vi "Field Draw Field(circular).vi"(7 "FieldRef":refnum<class "Field.lvclass">=refnum, 8 "new picture in":picture, 9 "Offset":cluster{"Width":dbl, "Height":dbl}, 10 "Scale":dbl) -> (0 "new picture out":picture, 1 "Offset Out":cluster{"Width":dbl, "Height":dbl}, 2 "Scale Out":dbl)   [LabVIEW 2022 SP3]
uses:
  Field_class/Field.lvclass
panel:
  in  "left":i16=1
  in  "rect":T1
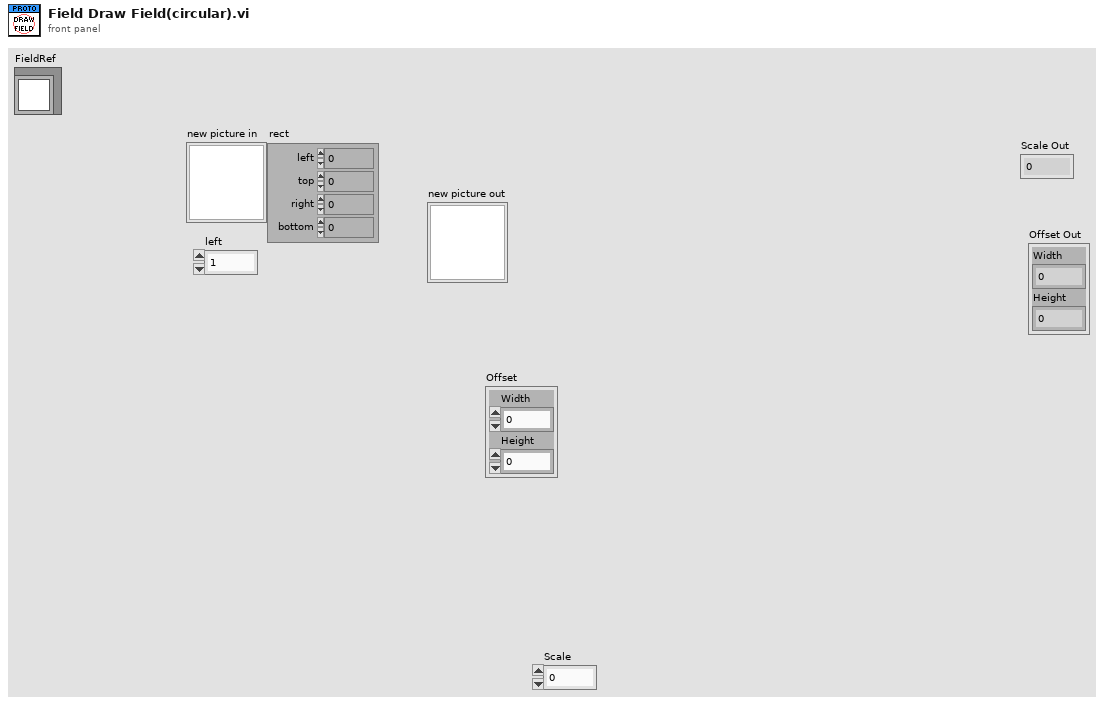
[diagram p1: front panel]
types:
  T1 = cluster{"left":i16, "top":i16, "right":i16, "bottom":i16}
  T2 = cluster{"Width":i16, "Style":enum32{"Solid", "Dash", "Dot", "DashDot", "DashDotDot"}}
  T3 = cluster{"boundary_width":i32, "center_circle_radius":i32, "defense_stretch":i32, "defense_width_or_radius":i32, "field_length":i32, "field_width":i32, "free_kick_from_defense_dist":i32, "goal_depth":i32, "goal_wall_width":i32, "goal_width":i32, "line_width":i32, "penalty_line_from_spot_dist":i32, "penalty_spot_from_field_line_dist":i32, "referee_width":i32}
  T4 = cluster{"boundary_width":dbl, "center_circle_radius":dbl, "defense_stretch":dbl, "defense_width_or_radius":dbl, "field_length":dbl, "field_width":dbl, "free_kick_from_defense_dist":dbl, "goal_depth":dbl, "goal_wall_width":dbl, "goal_width":dbl, "line_width":dbl, "penalty_line_from_spot_dist":dbl, "penalty_spot_from_field_line_dist":dbl, "referee_width":dbl}
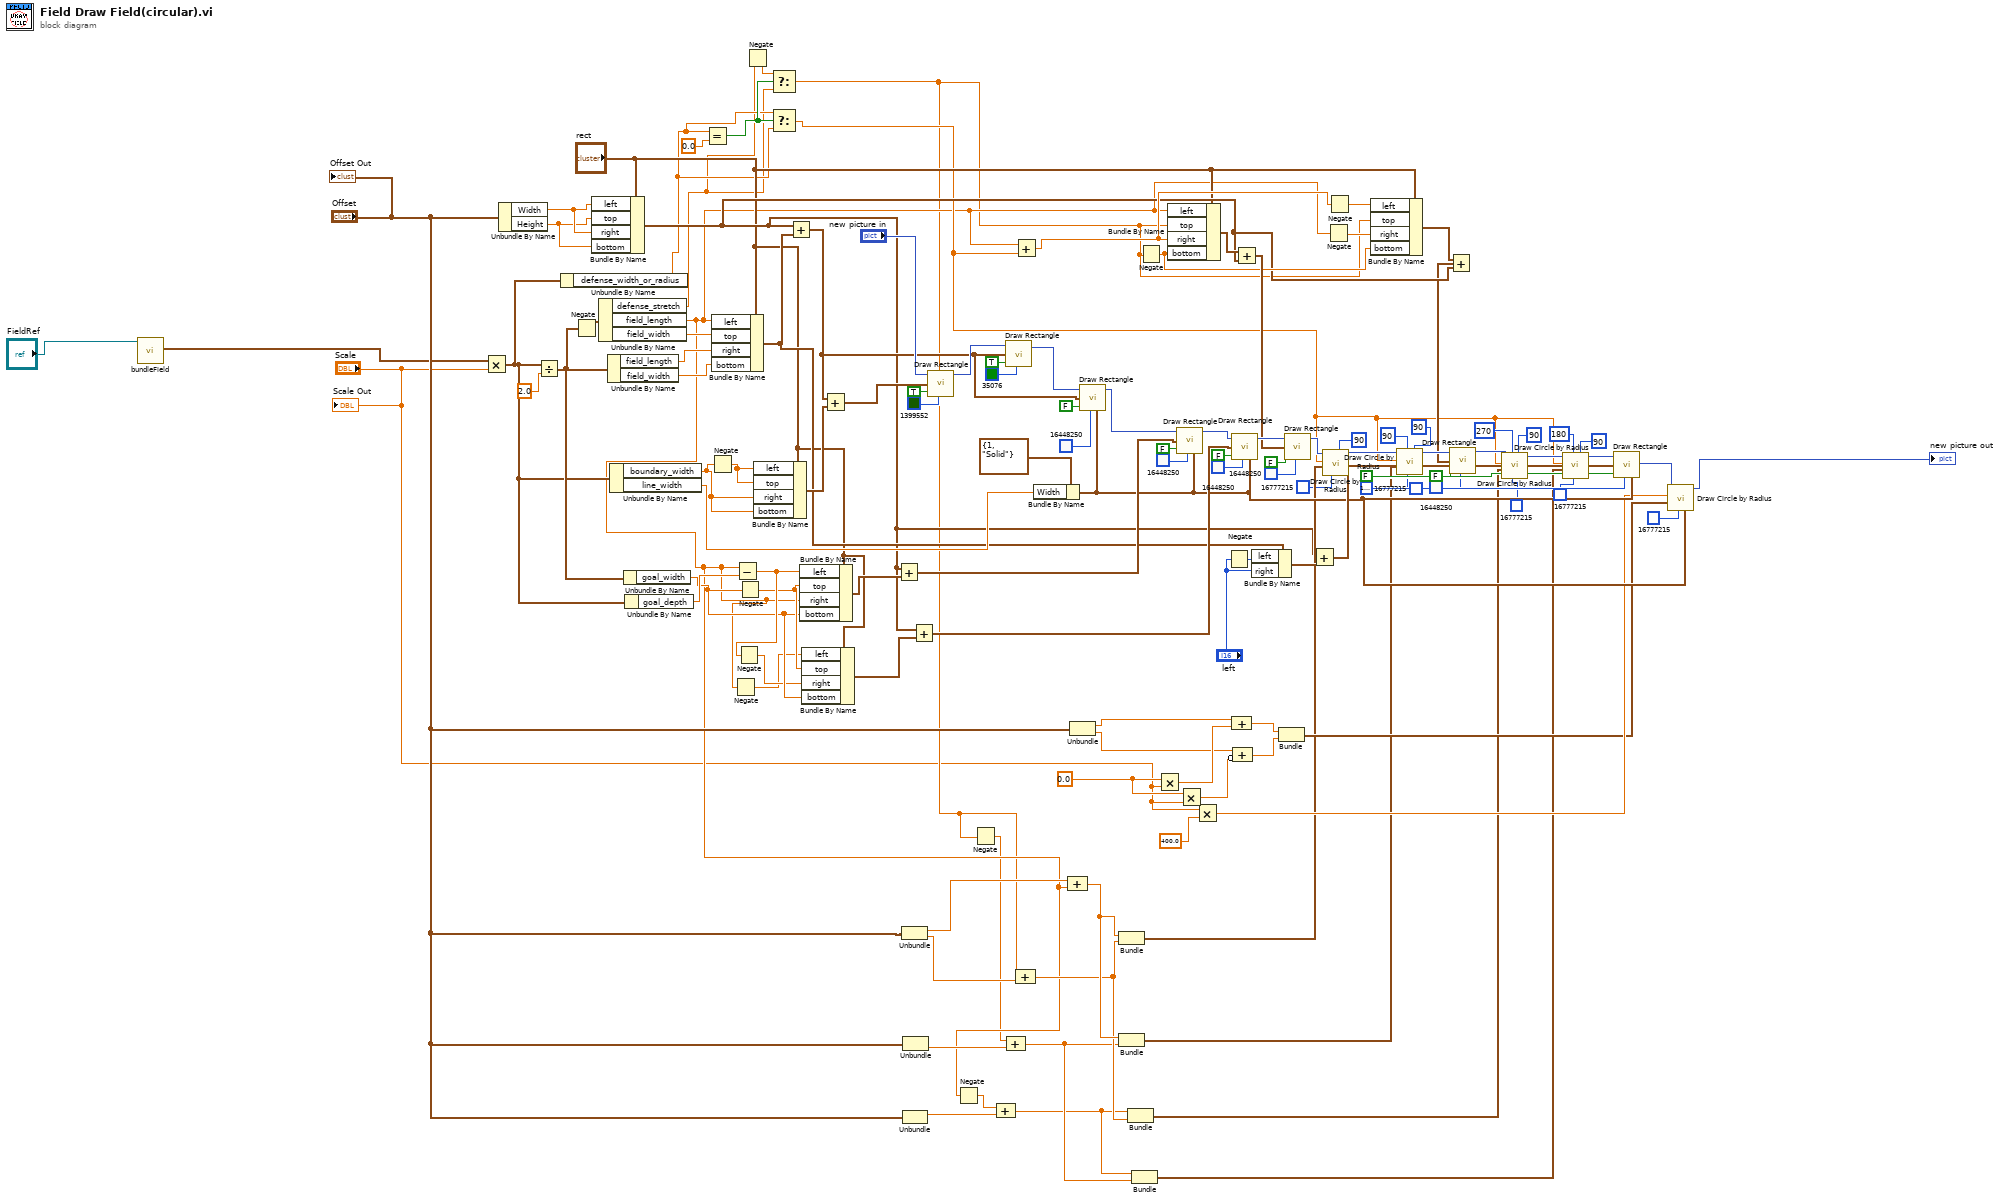
[diagram p0: block diagram]
diagram:
  w60 = 0.0 ("x")
  n1 = call "bundleField.vi"("Field in"="FieldRef") -> ("Cluster"=w3:T3)  [unwired: 8 in, 2 out]
  n2 = Multiply(x=w3, y="Scale") -> (x*y=w59:T4)
  n3 = Unbundle By Name("Offset") -> ("Width"=w117:dbl, "Height"=w116:dbl)
  n4 = Divide(x=w59, y=2.0) -> (x/y=w92:T4)
  n5 = Unbundle By Name(w59) -> ("defense_width_or_radius"=w2:dbl)
  n6 = Negate(x=w92) -> (-x=w112:T4)
  n7 = Bundle By Name(cluster="rect", "left"=w117, "top"=w116, "right"=w117, "bottom"=w116) -> (w33:T1)
  n8 = Unbundle By Name(w112) -> ("defense_stretch"=w1:dbl, "field_length"=w9:dbl, "field_width"=w115:dbl)
  n9 = Unbundle By Name(w92) -> ("field_length"=w114:dbl, "field_width"=w113:dbl)
  n10 = Unbundle By Name(w59) -> ("boundary_width"=w110:dbl, "line_width"=w99:dbl)
  n11 = Unbundle By Name(w92) -> ("goal_width"=w86:dbl)
  n12 = Unbundle By Name(w59) -> ("goal_depth"=w91:dbl)
  n13 = Equal?(x=w2, y=0.0) -> (x = y?=w11:bool)
  n14 = Negate(x=w110) -> (-x=w111:dbl)
  n15 = Bundle By Name(cluster="rect", "left"=w9, "top"=w115, "right"=w114, "bottom"=w113) -> (w79:T1)
  n16 = Negate(x=w9) -> (-x=w82:dbl)
  n17 = Subtract(x=w9, y=w91) -> (x-y=w88:dbl)
  n18 = Negate(x=w88) -> (-x=w83:dbl)
  n19 = Negate(x=w86) -> (-x=w87:dbl)
  n20 = Negate(x=w1) -> (-x=w6:dbl)
  n21 = Bundle By Name(cluster="rect", "left"=w111, "top"=w111, "right"=w110, "bottom"=w110) -> (w109:T1)
  n22 = Select(t=w6, s=w11, f=w1) -> (s? t:f=w8:dbl)
  n23 = Select(t=w2, s=w11, f=w2) -> (s? t:f=w10:dbl)
  n24 = Add(x=w33, y=w79) -> (x+y=w70:T1)
  n25 = Bundle By Name(cluster="rect", "left"=w88, "top"=w87, "right"=w9, "bottom"=w86) -> (w90:T1)
  n26 = Bundle By Name(cluster="rect", "left"=w82, "top"=w87, "right"=w83, "bottom"=w86) -> (w85:T1)
  n27 = Add(x=w70, y=w109) -> (x+y=w105:T1)
  n28 = Add(x=w33, y=w90) -> (x+y=w89:T1)
  n29 = Unbundle("Offset") -> ("Width"=w53:dbl, "Height"=w52:dbl)
  n30 = Unbundle("Offset") -> ("Width"=w16:dbl)  [unwired: 1 out]
  n31 = Unbundle("Offset") -> ("Height"=w47:dbl)  [unwired: 1 out]
  n32 = Add(x=w33, y=w85) -> (x+y=w84:T1)
  n33 = call <vilib>:"Draw Rectangle.vi"("picture"="new picture in", "rect"=w105, "fill?(F)"=TRUE, "color(black)"=u32 1399552) -> ("new picture"=w104:picture)  [unwired: 5 in]
  n34 = Negate(x=w9) -> (-x=w15:dbl)
  n35 = Negate(x=w8) -> (-x=w7:dbl)
  n36 = Compound Arithmetic op=ADD(w15, w16) -> (w13:dbl)
  n37 = call <vilib>:"Draw Rectangle.vi"("picture"=w104, "rect"=w70, "fill?(F)"=TRUE, "color(black)"=u32 35076) -> ("new picture"=w101:picture)  [unwired: 5 in]
  n38 = Compound Arithmetic op=ADD(w7, w47) -> (w17:dbl)
  n39 = Add(x=w9, y=w10) -> (x+y=w40:dbl)
  n40 = Compound Arithmetic op=ADD(w8, w52) -> (w24:dbl)
  n41 = Bundle By Name(cluster=T2 {"Width"=1, "Style"=enum."Solid"} ("pen"), "Width"=w99) -> (w72:T2)
  n42 = Compound Arithmetic op=ADD(w53, w9) -> (w30:dbl)
  n43 = Unbundle("Offset") -> ("Width"=w68:dbl, "Height"=w65:dbl)
  n44 = call <vilib>:"Draw Rectangle.vi"("picture"=w101, "rect"=w70, "fill?(F)"=FALSE, "color(black)"=u32 16448250, "pen"=w72) -> ("new picture"=w96:picture)  [unwired: 4 in]
  n45 = Bundle(w30, w24) -> (w51:cluster{dbl, dbl})  [unwired: 1 in]
  n46 = Bundle(w30, w17) -> (w44:cluster{dbl, dbl})  [unwired: 1 in]
  n47 = Bundle(w13, w24) -> (w28:cluster{dbl, dbl})  [unwired: 1 in]
  n48 = Bundle(w13, w17) -> (w23:cluster{dbl, dbl})  [unwired: 1 in]
  n49 = Negate(x=w8) -> (-x=w38:dbl)
  n50 = Multiply(x=w60, y="Scale") -> (x*y=w67:dbl)
  n51 = Bundle By Name(cluster="rect", "left"=w9, "top"=w8, "right"=w40, "bottom"=w38) -> (w55:T1)
  n52 = call <vilib>:"Draw Rectangle.vi"("picture"=w96, "rect"=w89, "fill?(F)"=FALSE, "color(black)"=u32 16448250, "pen"=w72) -> ("new picture"=w93:picture)  [unwired: 4 in]
  n53 = Multiply(x=w60, y="Scale") -> (x*y=w64:dbl)
  n54 = Multiply(x="Scale", y=sgl 400.0 ("radius")) -> (x*y=w62:dbl)
  n55 = Negate(x="left") -> (-x=w75:i16)
  n56 = call <vilib>:"Draw Rectangle.vi"("picture"=w93, "rect"=w84, "fill?(F)"=FALSE, "color(black)"=u32 16448250, "pen"=w72) -> ("new picture"=w56:picture)  [unwired: 4 in]
  n57 = Compound Arithmetic op=ADD(w68, w67) -> (w66:dbl)
  n58 = Compound Arithmetic op=ADD(w65, invert w64) -> (w63:dbl)
  n59 = Add(x=w55, y=w33) -> (x+y=w54:T1)
  n60 = Bundle By Name(cluster=w79, "left"=w75, "right"="left") -> (w78:T1)
  n61 = Bundle(w66, w63) -> (w61:cluster{dbl, dbl})  [unwired: 1 in]
  n62 = call <vilib>:"Draw Rectangle.vi"("picture"=w56, "rect"=w54, "fill?(F)"=FALSE, "color(black)"=u32 16448250) -> ("new picture"=w49:picture)  [unwired: 5 in]
  n63 = Add(x=w33, y=w78) -> (x+y=w77:T1)
  n64 = call <vilib>:"Draw Circle by Radius.vi"("arc size(360)"=i16 90, "color(black)"=u32 16777215, "pixel center"=w51, "radius"=w10, "picture"=w49) -> ("new picture"=w46:picture)  [unwired: 6 in]
  n65 = Negate(x=w9) -> (-x=w41:dbl)
  n66 = Negate(x=w40) -> (-x=w39:dbl)
  n67 = Bundle By Name(cluster="rect", "left"=w39, "top"=w8, "right"=w41, "bottom"=w38) -> (w34:T1)
  n68 = call <vilib>:"Draw Circle by Radius.vi"("arc size(360)"=i16 90 ("start angle(0)"), "color(black)"=u32 16777215, "start angle(0)"=i16 90, "pixel center"=w44, "radius"=w10, "picture"=w46) -> ("new picture"=w35:picture)  [unwired: 5 in]
  n69 = Add(x=w34, y=w33) -> (x+y=w32:T1)
  n70 = call <vilib>:"Draw Rectangle.vi"("picture"=w35, "rect"=w32, "fill?(F)"=FALSE, "color(black)"=u32 16448250) -> ("new picture"=w29:picture)  [unwired: 5 in]
  n71 = call <vilib>:"Draw Circle by Radius.vi"("arc size(360)"=i16 90, "color(black)"=u32 16777215, "start angle(0)"=i16 270, "pixel center"=w28, "radius"=w10, "picture"=w29) -> ("new picture"=w21:picture)  [unwired: 5 in]
  n72 = call <vilib>:"Draw Circle by Radius.vi"("arc size(360)"=i16 90, "color(black)"=u32 16777215, "start angle(0)"=i16 180, "pixel center"=w23, "radius"=w10, "picture"=w21) -> ("new picture"=w20:picture)  [unwired: 5 in]
  n73 = call <vilib>:"Draw Rectangle.vi"("picture"=w20, "rect"=w77, "fill?(F)"=FALSE, "color(black)"=u32 16777226, "pen"=w72) -> ("new picture"=w74:picture)  [unwired: 4 in]
  n74 = call <vilib>:"Draw Circle by Radius.vi"("pen"=w72, "color(black)"=u32 16777215, "pixel center"=w61, "radius"=w62, "picture"=w74) -> ("new picture"=→"new picture out":picture)  [unwired: 6 in]
  "Scale Out" <- "Scale"
  "Offset Out" <- "Offset"
